vi "hackrf_spectrum_analyser.vi"() -> ()   [LabVIEW 2020]
doc: "Demonstrates how to open a connection to an TCP server, read the data being sent, and display the data on a chart. This VI is designed to stop if the TCP connection is terminated."
panel:
  in  "Apply":bool
  in  "Max, MHz":dbl format="%#_4g"
  in  "Min, MHz":dbl format="%#_4g"
  out "XY Graph":cluster{"Y":dbl[], "Y":dbl[]}[](graph)
  in  "Server IPv4 Address":string
  in  "Server TCP Port":dbl
  in  "Server Closed":string="The server VI closed the connection."
  in  "Stop":bool
  # "Overview: Demonstrates the use of the TCP functions to connect to a TCP server VI and receive data.\nInstructions:\n1. Ensure Simple TCP - Server.vi is already running.\n2. Run the VI.\n3. Click Stop to stop the VI. Note that if you stop the server VI, this VI will stop automatically."
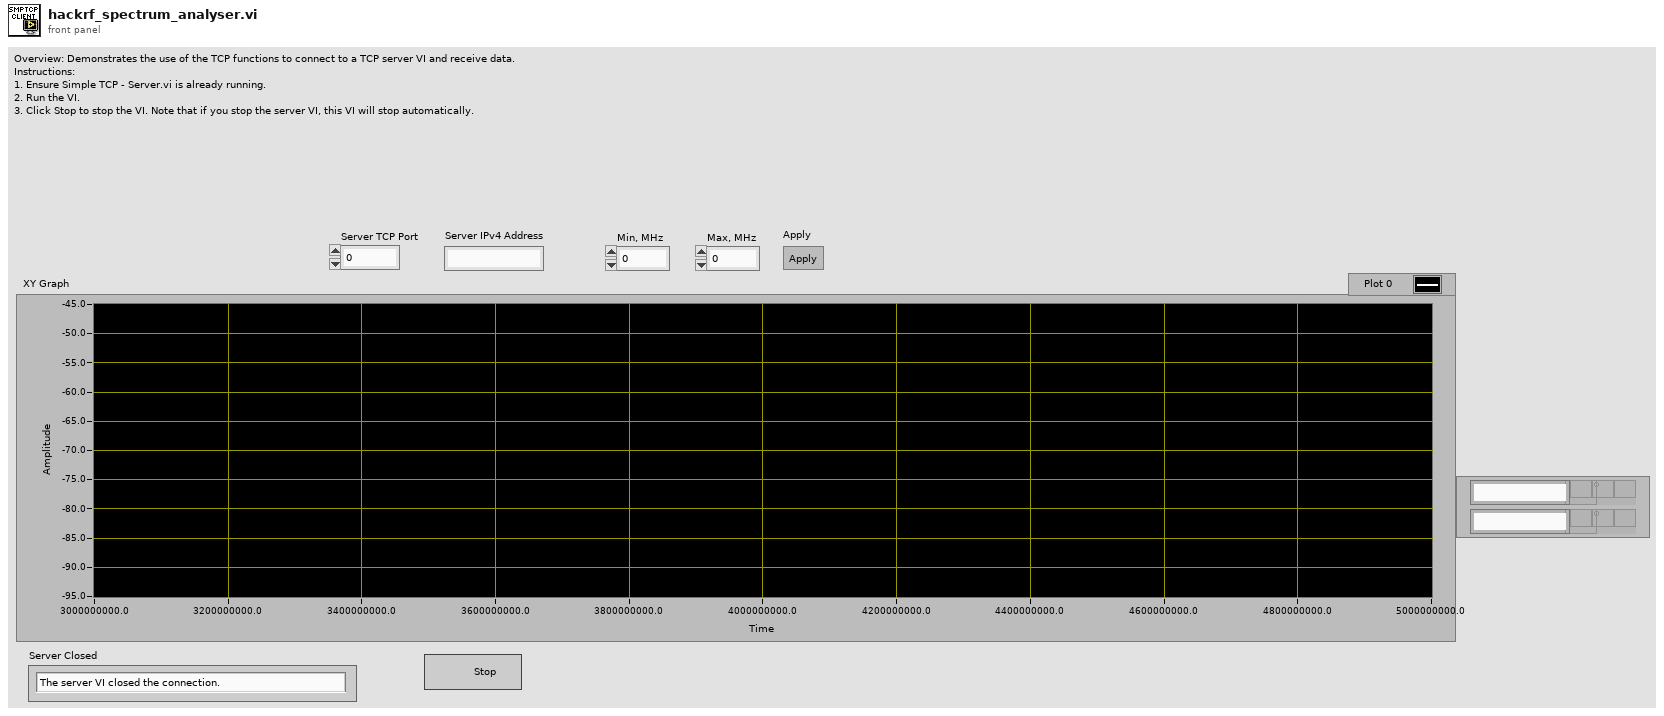
[diagram p1: front panel]
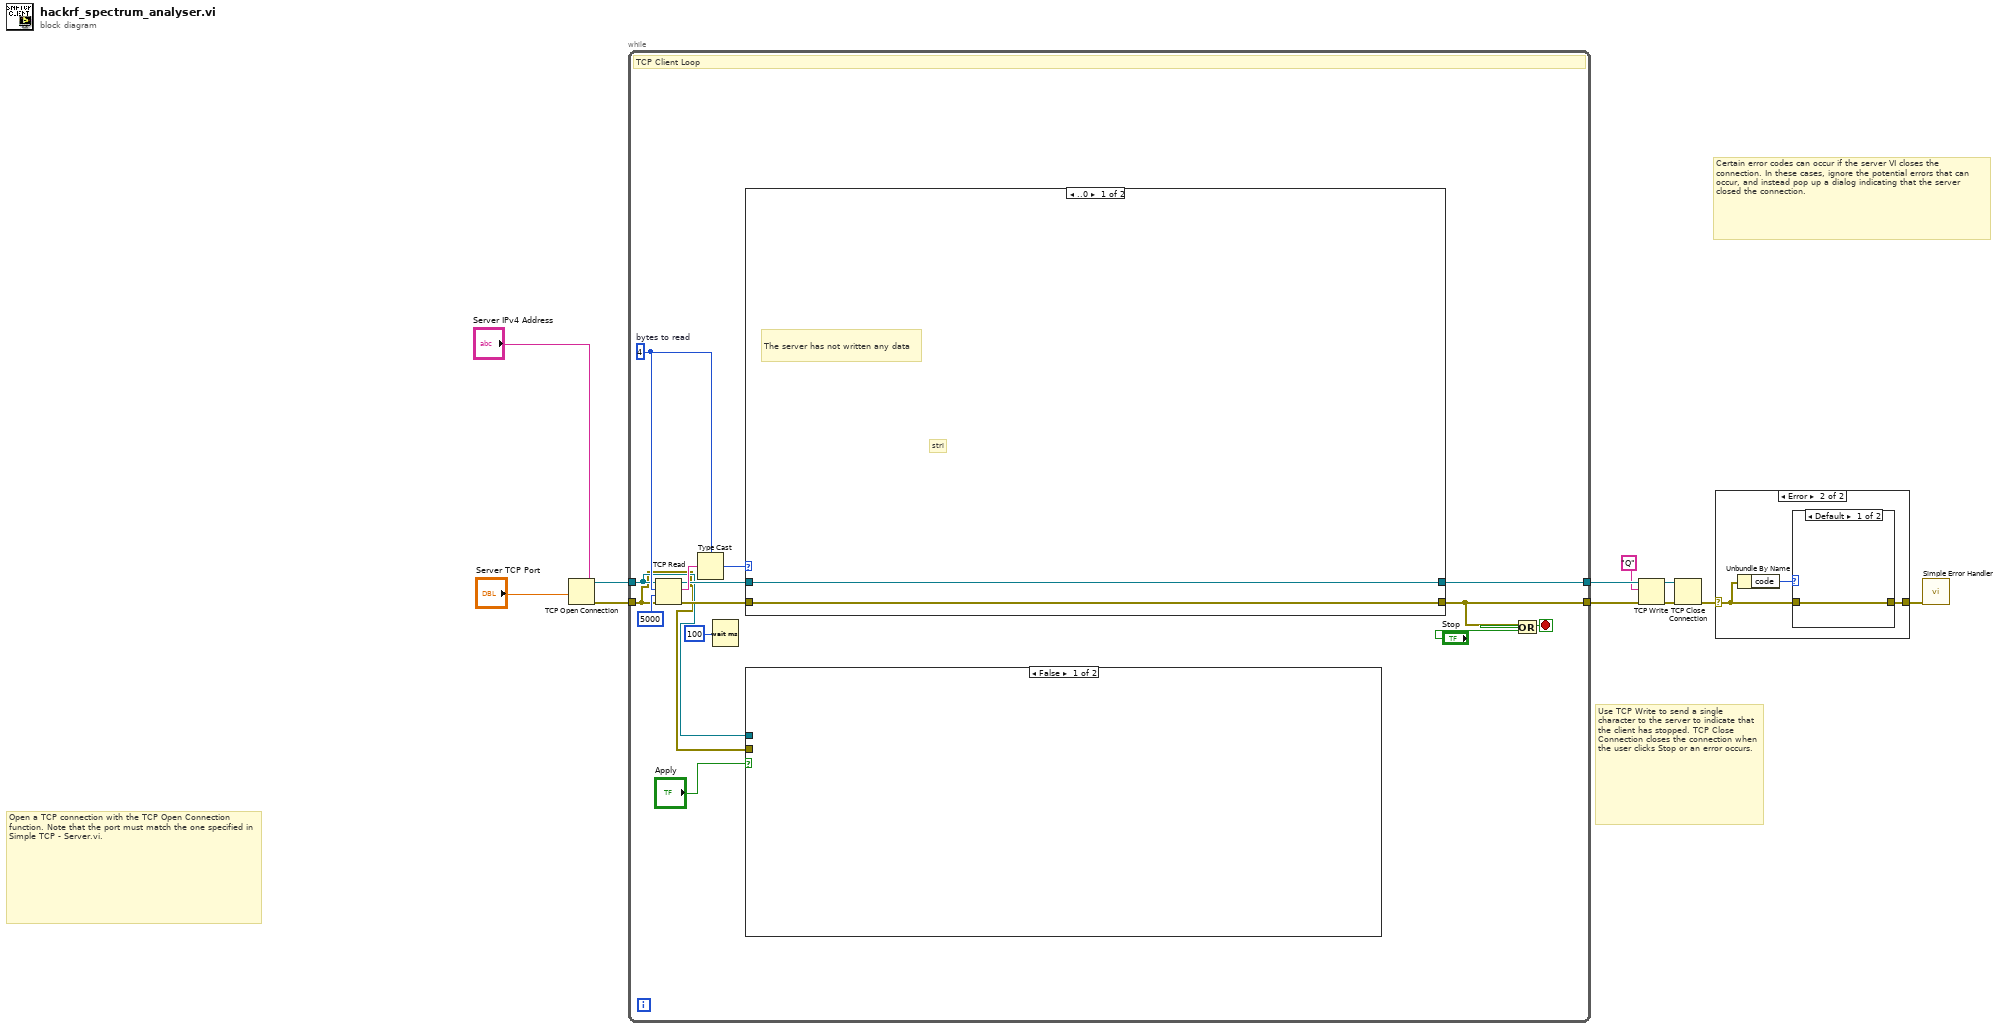
[diagram p0: block diagram]
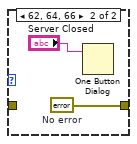
[diagram p3: hidden frame]
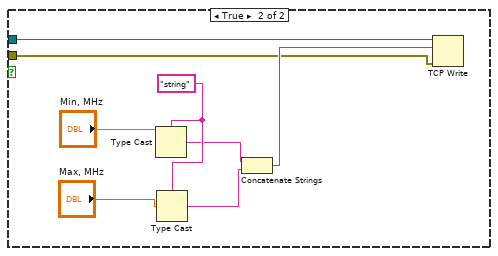
[diagram p4: hidden frame]
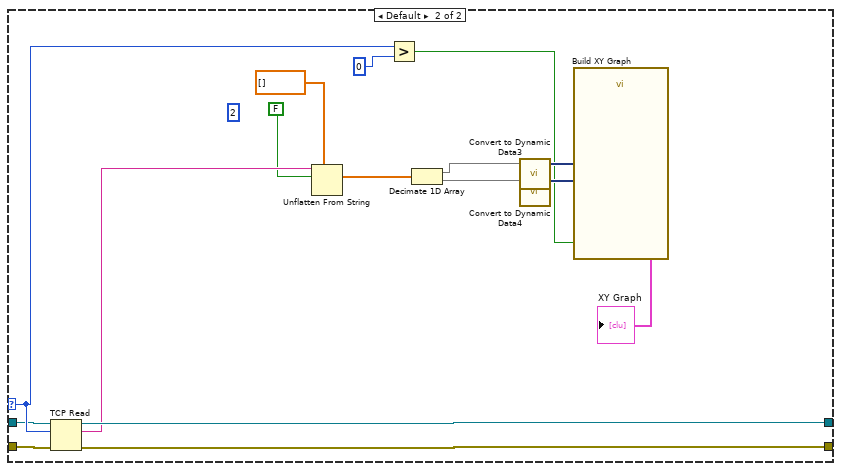
[diagram p5: hidden frame]
diagram:
  # "Certain error codes can occur if the server VI closes the connection. In these cases, ignore the potential errors that can occur, and instead pop up a dialog indicating that the server closed the connection."
  # "Use TCP Write to send a single character to the server to indicate that the client has stopped. TCP Close Connection closes the connection when the user clicks Stop or an error occurs."
  # "Open a TCP connection with the TCP Open Connection function. Note that the port must match the one specified in Simple TCP - Server.vi."
  n1 = TCP Open Connection(address="Server IPv4 Address", remote port or service name="Server TCP Port") -> (connection ID=w2:refnum<k5>, error out=w1:errorcluster)  [unwired: 3 in]
  n2 = while {
    tunnel: w1 -> [w13]
    tunnel: w2 -> [w14]
    tunnel: [w18] -> w10
    tunnel: [w17] -> w8
    stop <- w20 stop-if-true
    w22 = 4  # bytes to read
    # "TCP Client Loop"
    n3 = TCP Read(connection ID=w14, bytes to read=w22, error in (no error)=w13, 9:5000 ("timeout ms (25000)")) -> (connection ID out=w24:refnum<k5>, data out=w25:string, error out=w23:errorcluster)  [unwired: 1 in]
    n4 = Type Cast(type=w22, x=w25) -> (*(type *) &x=w16:i32)
    n5 = Wait (ms)(milliseconds to wait=u32 100) -> ()  [unwired: 1 out]
    n6 = case shown="..0" w16 {
      selector: w16 -> [_ w42]
      tunnel: w24 -> [w35 w36]
      tunnel: w23 -> [w34 w51]
      tunnel: [w35 w50] -> w18
      tunnel: [w34 w49] -> w17
      frame ..0 {
        # "stri"
        # "The server has not written any data"
      }
      frame Default {
        (unwired) 2
        n7 = TCP Read(connection ID=w36, bytes to read=w42, error in (no error)=w51) -> (connection ID out=w50:refnum<k5>, data out=w48:string, error out=w49:errorcluster)  [unwired: 2 in]
        n8 = Unflatten From String(type=dbl[] [] ("chart"), binary string=w48, data includes array or string size? (T)=FALSE) -> (value=w46:dbl[])  [unwired: 2 in, 2 out]
        n9 = Greater?(x=w42, y=0) -> (0:w37:bool)
        n10 = Decimate 1D Array(w46) -> (w41:dbl[], w39:dbl[])
        n11 = call "Convert to Dynamic Data3"("Array"=w41) -> ("Dynamic Data Type"=w40:dynamicdata)  [unwired: 3 in]
        n12 = call "Convert to Dynamic Data4"("Array"=w39) -> ("Dynamic Data Type"=w38:dynamicdata)  [unwired: 3 in]
        n13 = call "Build XY Graph"("Reset"=w37, "Y Input"=w38, "X Input"=w40) -> ("XY Graph"=→"XY Graph":cluster{"Y":dbl[], "Y":dbl[]}[])  [unwired: 2 in, 6 out]
      }
    }
    n14 = case shown="False" "Apply" {
      tunnel: w14 -> [_ w33]
      tunnel: w13 -> [_ w31]
      frame False {
      }
      frame True {
        w30 = "string"
        n15 = Type Cast(type=w30, x="Min, MHz") -> (*(type *) &x=w26:string)
        n16 = Type Cast(type=w30, x="Max, MHz") -> (*(type *) &x=w27:string)
        n17 = Concatenate Strings(w26, w27) -> (w32:string)
        n18 = TCP Write(connection ID=w33, data in=w32, error in (no error)=w31) -> ()  [unwired: 4 out]
      }
    }
    n19 = Or(x=w17, y="Stop") -> (x .or. y?=w20:bool)
  }
  n20 = TCP Write(connection ID=w10, data in="Q", error in (no error)=w8) -> (connection ID out=w11:refnum<k5>, error out=w9:errorcluster)  [unwired: 2 out]
  n21 = TCP Close Connection(connection ID=w11, error in (no error)=w9) -> (error out=w6:errorcluster)  [unwired: 1 in, 1 out]
  n22 = case shown="Error" w6 {
    selector: w6 -> [w52 w54]
    tunnel: [w52 w53] -> w5
    frame No Error {
    }
    frame Error {
      n23 = Unbundle By Name(w54) -> ("code"=w55:i32)
      n24 = case shown="Default" w55 {
        tunnel: w54 -> [w56 _]
        tunnel: [w56 w58] -> w53
        frame Default {
        }
        frame 62, 64, 66 {
          w58 = errorcluster {"status"=FALSE, "code"=0, "source"=""}  # No error
          n25 = One Button Dialog(message="Server Closed") -> ()  [unwired: 1 in, 1 out]
        }
      }
    }
  }
  n26 = call <vilib>:"Simple Error Handler.vi"("error in (no error)"=w5) -> ()  [unwired: 4 in, 5 out]
